vi "converter.vi"(5 "On/Off":bool=TRUE, 6 "Error In":errorcluster, 8 "Digit":u8) -> (0 "Error Out":errorcluster, 2 "Digit":T1)   [LabVIEW 2012]
uses:
  black bg digit.ctl
  vertical.ctl
  horizontal.ctl
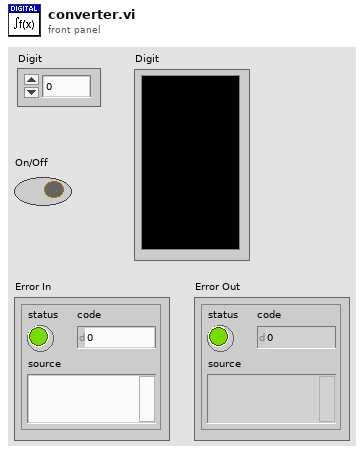
[diagram p1: front panel]
types:
  T1 = typedef "black bg digit.ctl" = cluster{"V1":T2, "V2":T2, "H1":T3, "H2":T3, "V3":T2, "V4":T2, "H3":T3}
  T2 = typedef "vertical.ctl" = bool
  T3 = typedef "horizontal.ctl" = bool
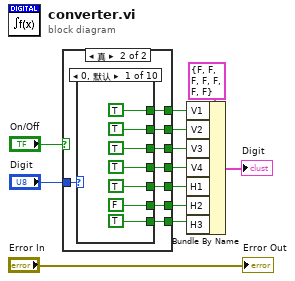
[diagram p0: block diagram]
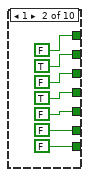
[diagram p3: hidden frame]
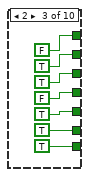
[diagram p4: hidden frame]
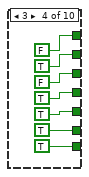
[diagram p5: hidden frame]
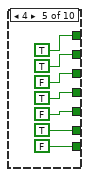
[diagram p6: hidden frame]
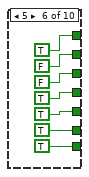
[diagram p7: hidden frame]
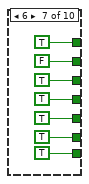
[diagram p8: hidden frame]
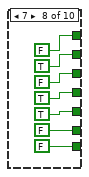
[diagram p9: hidden frame]
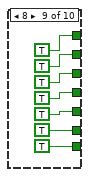
[diagram p10: hidden frame]
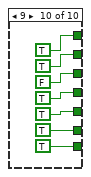
[diagram p11: hidden frame]
diagram:
  n1 = case shown="真" "On/Off" {
    tunnel: "Digit" -> [_ w20]
    tunnel: [_ w19] -> w11
    tunnel: [_ w18] -> w10
    tunnel: [_ w17] -> w9
    tunnel: [_ w16] -> w8
    tunnel: [_ w15] -> w7
    tunnel: [_ w14] -> w6
    tunnel: [_ w13] -> w5
    frame False {
    }
    frame True {
      n2 = case shown="0, 默认" w20 {
        tunnel: [TRUE FALSE FALSE FALSE TRUE TRUE TRUE FALSE TRUE TRUE] -> w19
        tunnel: [TRUE TRUE TRUE TRUE TRUE FALSE FALSE TRUE TRUE TRUE] -> w18
        tunnel: [TRUE FALSE TRUE FALSE FALSE FALSE TRUE FALSE TRUE FALSE] -> w17
        tunnel: [TRUE TRUE FALSE TRUE TRUE TRUE TRUE TRUE TRUE TRUE] -> w16
        tunnel: [TRUE FALSE TRUE TRUE FALSE TRUE TRUE TRUE TRUE TRUE] -> w15
        tunnel: [FALSE FALSE TRUE TRUE TRUE TRUE TRUE FALSE TRUE TRUE] -> w14
        tunnel: [TRUE FALSE TRUE TRUE FALSE TRUE TRUE FALSE TRUE TRUE] -> w13
        frame 0, Default {
        }
        frame 1 {
        }
        frame 2 {
        }
        frame 3 {
        }
        frame 4 {
        }
        frame 5 {
        }
        frame 6 {
        }
        frame 7 {
        }
        frame 8 {
        }
        frame 9 {
        }
      }
    }
  }
  n3 = Bundle By Name(cluster=T1 {"V1"=FALSE, "V2"=FALSE, "H1"=FALSE, "H2"=FALSE, "V3"=FALSE, "V4"=FALSE, "H3"=FALSE} ("Digit 2"), "V1"=w11, "V2"=w10, "V3"=w9, "V4"=w8, "H1"=w7, "H2"=w6, "H3"=w5) -> (→"Digit":T1)
  "Error Out" <- "Error In"
